vi "PeakDetect_FilterMinimumPeakWidth.vi"(6 "minimumPeakWidth":dbl format="%#_13g", 8 "Error In":errorcluster, 11 "Peak Info In":T1[](array[typedef])) -> (0 "Error Out":errorcluster, 3 "Peak Info Out":T1[](array[typedef]))   [LabVIEW 2015]
uses:
  Controls/PeakInfoPresenter.ctl
panel:
  in  "MinimumSlopeToUsePeakMax":dbl format="%#_13g"
  in  "Intensities":dbl[](array[numeric])=[55.0, 56.0, 46.0, 32.0, 21.0, 37.0, 92.0, 179.0, 213.0, 312.0, 312.0, 297.0, 296.0, 224.0, 192.0, 50.0, 58.0, 96.0, 112.0, 108.0, 107.0, 117.0, 101.0, 79.0, 28.0, 242.0, 3002.0, 4321.0, 6382.0, 8039.0, 8112.0, 7467.0, 6673.0, 6730.0, 4821.0, 161.0, 116.0, 199.0, 280.0, 324.0, 385.0, 306.0, 340.0, 270.0, 209.0, 596.0, 8839.0, 15018.0, 22096.0, 27306.0, 28282.0, 26382.0, 24772.0, 19971.0, 16031.0, 677.0, 291.0, 595.0, 848.0, 1124.0, 1192.0, 1040.0, 1069.0, 767.0, 821.0, 50.0, 66.0, 105.0, 160.0, 163.0, 147.0, 163.0, 127.0, 96.0, 73.0, 9.0, 4.0, 4.0, 19.0, 10.0, 14.0, 8.0, 14.0, 7.0, 9.0, 44.0, 57.0, 86.0, 126.0, 111.0, 98.0, 79.0, 95.0, 67.0, 16.0, 19.0, 17.0, 25.0, 30.0, 39.0, 38.0, 191.0, 275.0, 254.0, 270.0, 293.0, 216.0, 219.0, 170.0, 180.0, 186.0, 212.0, 255.0, 355.0, 365.0, 354.0, 352.0, 389.0, 310.0, 272.0, 208.0, 189.0, 175.0, 203.0, 226.0, 202.0, 206.0, 278.0, 279.0, 414.0, 799.0, 1517.0, 2446.0, 3938.0, 4796.0, 5265.0, 5583.0, 5257.0, 4438.0, 3543.0, 2831.0, 1347.0, 1119.0, 1370.0, 1782.0, 1807.0, 1828.0, 2082.0, 2011.0, 2473.0, 4735.0, 8059.0, 13114.0, 21491.0, 25990.0, 28670.0, 29595.0, 29953.0, 26733.0, 21472.0, 14896.0, 7745.0, 6381.0, 7465.0, 9646.0, 10328.0, 10403.0, 10136.0, 9622.0, 7344.0, 5462.0, 2287.0, 1703.0, 2115.0, 2635.0, 3263.0, 4044.0, 5060.0, 5508.0, 6042.0, 6139.0, 6124.0, 6909.0, 7394.0, 6919.0, 6393.0, 5036.0, 5125.0, 4926.0, 3939.0, 3280.0, 2071.0, 2019.0, 1927.0, 1569.0, 1324.0, 992.0, 958.0, 880.0, 889.0, 993.0, 1241.0, 163.0, 122.0, 143.0, 189.0, 188.0, 214.0, 226.0, 254.0, 230.0, 216.0, 170.0, 164.0, 205.0, 153.0, 204.0, 137.0, 171.0, 163.0, 229.0, 313.0, 468.0, 667.0, 1041.0, 1532.0, 1899.0, 2343.0, 2797.0, 2956.0, 2591.0, 1993.0, 1475.0, 787.0, 702.0, 842.0, 1073.0, 1341.0, 1708.0, 1886.0, 2506.0, 3796.0, 5659.0, 7754.0, 13596.0, 19036.0, 25687.0, 30761.0, 35888.0, 37967.0, 35251.0, 27029.0, 21428.0, 11593.0, 9040.0, 11127.0, 13005.0, 16089.0, 18097.0, 19329.0, 19088.0, 14510.0, 10053.0, 6086.0, 4080.0, 4322.0, 4947.0, 5697.0, 6188.0, 6839.0, 6325.0, 5298.0, 3850.0, 2157.0, 1592.0, 1569.0, 1697.0, 1935.0, 1994.0, 2079.0, 2043.0, 1563.0, 1245.0, 826.0, 516.0, 585.0, 620.0, 609.0, 625.0, 651.0, 677.0, 707.0, 761.0, 879.0, 1091.0, 1597.0, 1813.0, 2074.0, 2314.0, 2176.0, 2032.0, 1570.0, 1155.0, 21.0, 18.0, 5.0, 22.0, 10.0, 11.0, 23.0, 8.0, 11.0, 20.0, 14.0, 12.0, 22.0, 8.0, 12.0, 19.0, 14.0, 16.0, 9.0, 18.0, 12.0, 21.0, 16.0, 22.0, 13.0, 20.0, 13.0, 26.0, 26.0, 44.0, 30.0, 56.0, 52.0, 39.0, 33.0, 26.0, 18.0, 29.0, 34.0, 36.0, 39.0, 47.0, 55.0, 113.0, 124.0, 202.0, 279.0, 355.0, 573.0, 856.0, 1150.0, 1298.0, 1700.0, 1791.0, 1294.0, 1052.0, 874.0, 526.0, 667.0, 865.0, 992.0, 1286.0, 1427.0, 1381.0, 1239.0, 962.0, 662.0, 386.0, 392.0, 452.0, 513.0, 627.0, 706.0, 779.0, 523.0, 425.0, 309.0, 188.0, 172.0, 182.0, 179.0, 207.0, 285.0, 246.0, 231.0, 183.0, 112.0, 65.0, 58.0, 81.0, 73.0, 95.0, 110.0, 112.0, 67.0, 78.0, 79.0, 70.0, 78.0, 92.0, 108.0, 43.0, 40.0, 52.0, 32.0, 53.0, 51.0, 37.0, 35.0, 43.0, 33.0, 39.0, 48.0, 62.0, 38.0, 40.0, 31.0, 42.0, 31.0, 47.0, 41.0, 41.0, 46.0, 49.0, 59.0, 49.0, 56.0, 66.0, 49.0, 57.0, 78.0, 107.0, 139.0, 196.0, 263.0, 350.0, 506.0, 639.0, 850.0, 963.0, 1256.0, 1355.0, 1989.0, 2163.0, 2256.0, 2168.0, 2097.0, 1936.0, 1771.0, 1572.0, 1549.0, 1669.0, 1962.0, 1928.0, 2150.0, 2282.0, 1774.0, 1693.0, 1455.0, 1325.0, 1034.0, 984.0, 993.0, 1120.0, 1284.0, 1002.0, 1042.0, 931.0, 781.0, 614.0, 482.0, 424.0, 448.0, 432.0, 435.0, 521.0, 427.0, 389.0, 344.0, 261.0, 187.0, 173.0, 188.0, 218.0, 209.0, 195.0, 185.0, 181.0, 196.0, 212.0, 193.0, 240.0, 203.0, 266.0, 287.0, 280.0, 229.0, 230.0, 207.0, 196.0, 189.0, 180.0, 4.0, 10.0, 7.0, 13.0, 5.0, 15.0, 7.0, 3.0, 13.0, 8.0, 7.0, 8.0, 4.0, 12.0, 11.0, 4.0, 4.0, 11.0, 4.0, 6.0, 8.0, 1.0, 9.0, 11.0, 9.0, 7.0, 8.0, 16.0, 10.0, 13.0, 4.0, 6.0, 10.0, 10.0, 11.0, 15.0, 7.0, 9.0, 6.0, 7.0, 8.0, 16.0, 6.0, 12.0, 7.0, 16.0, 22.0, 63.0, 99.0, 111.0, 172.0, 250.0, 327.0, 379.0, 389.0, 354.0, 296.0, 269.0, 251.0, 177.0, 211.0, 221.0, 341.0, 372.0, 363.0, 332.0, 304.0, 314.0, 240.0, 145.0, 137.0, 169.0, 201.0, 238.0, 259.0, 183.0, 200.0, 192.0, 92.0, 77.0, 60.0, 91.0, 68.0, 87.0, 129.0, 90.0, 88.0, 76.0, 59.0, 28.0, 26.0, 22.0, 36.0, 33.0, 36.0, 47.0, 33.0, 41.0, 31.0, 38.0, 29.0]
  in  "Masses":dbl[](array[numeric])=[54.0, 54.1, 54.2, 54.3, 54.4, 54.5, 54.6, 54.7, 54.8, 54.9, 55.0, 55.1, 55.2, 55.3, 55.4, 55.5, 55.6, 55.7, 55.8, 55.9, 56.0, 56.1, 56.2, 56.3, 56.4, 56.5, 56.6, 56.7, 56.8, 56.9, 57.0, 57.1, 57.2, 57.3, 57.4, 57.5, 57.6, 57.7, 57.8, 57.9, 58.0, 58.1, 58.2, 58.3, 58.4, 58.5, 58.6, 58.7, 58.8, 58.9, 59.0, 59.1, 59.2, 59.3, 59.4, 59.5, 59.6, 59.7, 59.8, 59.9, 60.0, 60.1, 60.2, 60.3, 60.4, 60.5, 60.6, 60.7, 60.8, 60.9, 61.0, 61.1, 61.2, 61.3, 61.4, 61.5, 61.6, 61.7, 61.8, 61.9, 62.0, 62.1, 62.2, 62.3, 62.4, 62.5, 62.6, 62.7, 62.8, 62.9, 63.0, 63.1, 63.2, 63.3, 63.4, 63.5, 63.6, 63.7, 63.8, 63.9, 64.0, 611.0, 611.1, 611.2, 611.3, 611.4, 611.5, 611.6, 611.7, 611.8, 611.9, 612.0, 612.1, 612.2, 612.3, 612.4, 612.5, 612.6, 612.7, 612.8, 612.9, 613.0, 613.1, 613.2, 613.3, 613.4, 613.5, 613.6, 613.7, 613.8, 613.9, 614.0, 614.1, 614.2, 614.3, 614.4, 614.5, 614.6, 614.7, 614.8, 614.9, 615.0, 615.1, 615.2, 615.3, 615.4, 615.5, 615.6, 615.7, 615.8, 615.9, 616.0, 616.1, 616.2, 616.3, 616.4, 616.5, 616.6, 616.7, 616.8, 616.9, 617.0, 617.1, 617.2, 617.3, 617.4, 617.5, 617.6, 617.7, 617.8, 617.9, 618.0, 618.1, 618.2, 618.3, 618.4, 618.5, 618.6, 618.7, 618.8, 618.9, 619.0, 619.1, 619.2, 619.3, 619.4, 619.5, 619.6, 619.7, 619.8, 619.9, 620.0, 620.1, 620.2, 620.3, 620.4, 620.5, 620.6, 620.7, 620.8, 620.9, 621.0, 902.0, 902.1, 902.2, 902.3, 902.4, 902.5, 902.6, 902.7, 902.8, 902.9, 903.0, 903.1, 903.2, 903.3, 903.4, 903.5, 903.6, 903.7, 903.8, 903.9, 904.0, 904.1, 904.2, 904.3, 904.4, 904.5, 904.6, 904.7, 904.8, 904.9, 905.0, 905.1, 905.2, 905.3, 905.4, 905.5, 905.6, 905.7, 905.8, 905.9, 906.0, 906.1, 906.2, 906.3, 906.4, 906.5, 906.6, 906.7, 906.8, 906.9, 907.0, 907.1, 907.2, 907.3, 907.4, 907.5, 907.6, 907.7, 907.8, 907.9, 908.0, 908.1, 908.2, 908.3, 908.4, 908.5, 908.6, 908.7, 908.8, 908.9, 909.0, 909.1, 909.2, 909.3, 909.4, 909.5, 909.6, 909.7, 909.8, 909.9, 910.0, 910.1, 910.2, 910.3, 910.4, 910.5, 910.6, 910.7, 910.8, 910.9, 911.0, 911.1, 911.2, 911.3, 911.4, 911.5, 911.6, 911.7, 911.8, 911.9, 912.0, 1540.0, 1540.1, 1540.2, 1540.3, 1540.4, 1540.5, 1540.6, 1540.7, 1540.8, 1540.9, 1541.0, 1541.1, 1541.2, 1541.3, 1541.4, 1541.5, 1541.6, 1541.7, 1541.8, 1541.9, 1542.0, 1542.1, 1542.2, 1542.3, 1542.4, 1542.5, 1542.6, 1542.7, 1542.8, 1542.9, 1543.0, 1543.1, 1543.2, 1543.3, 1543.4, 1543.5, 1543.6, 1543.7, 1543.8, 1543.9, 1544.0, 1544.1, 1544.2, 1544.3, 1544.4, 1544.5, 1544.6, 1544.7, 1544.8, 1544.9, 1545.0, 1545.1, 1545.2, 1545.3, 1545.4, 1545.5, 1545.6, 1545.7, 1545.8, 1545.9, 1546.0, 1546.1, 1546.2, 1546.3, 1546.4, 1546.5, 1546.6, 1546.7, 1546.8, 1546.9, 1547.0, 1547.1, 1547.2, 1547.3, 1547.4, 1547.5, 1547.6, 1547.7, 1547.8, 1547.9, 1548.0, 1548.1, 1548.2, 1548.3, 1548.4, 1548.5, 1548.6, 1548.7, 1548.8, 1548.9, 1549.0, 1549.1, 1549.2, 1549.3, 1549.4, 1549.5, 1549.6, 1549.7, 1549.8, 1549.9, 1550.0, 1773.0, 1773.1, 1773.2, 1773.3, 1773.4, 1773.5, 1773.6, 1773.7, 1773.8, 1773.9, 1774.0, 1774.1, 1774.2, 1774.3, 1774.4, 1774.5, 1774.6, 1774.7, 1774.8, 1774.9, 1775.0, 1775.1, 1775.2, 1775.3, 1775.4, 1775.5, 1775.6, 1775.7, 1775.8, 1775.9, 1776.0, 1776.1, 1776.2, 1776.3, 1776.4, 1776.5, 1776.6, 1776.7, 1776.8, 1776.9, 1777.0, 1777.1, 1777.2, 1777.3, 1777.4, 1777.5, 1777.6, 1777.7, 1777.8, 1777.9, 1778.0, 1778.1, 1778.2, 1778.3, 1778.4, 1778.5, 1778.6, 1778.7, 1778.8, 1778.9, 1779.0, 1779.1, 1779.2, 1779.3, 1779.4, 1779.5, 1779.6, 1779.7, 1779.8, 1779.9, 1780.0, 1780.1, 1780.2, 1780.3, 1780.4, 1780.5, 1780.6, 1780.7, 1780.8, 1780.9, 1781.0, 1781.1, 1781.2, 1781.3, 1781.4, 1781.5, 1781.6, 1781.7, 1781.8, 1781.9, 1782.0, 1782.1, 1782.2, 1782.3, 1782.4, 1782.5, 1782.6, 1782.7, 1782.8, 1782.9, 1783.0, 1830.0, 1830.1, 1830.2, 1830.3, 1830.4, 1830.5, 1830.6, 1830.7, 1830.8, 1830.9, 1831.0, 1831.1, 1831.2, 1831.3, 1831.4, 1831.5, 1831.6, 1831.7, 1831.8, 1831.9, 1832.0, 1832.1, 1832.2, 1832.3, 1832.4, 1832.5, 1832.6, 1832.7, 1832.8, 1832.9, 1833.0, 1833.1, 1833.2, 1833.3, 1833.4, 1833.5, 1833.6, 1833.7, 1833.8, 1833.9, 1834.0, 1834.1, 1834.2, 1834.3, 1834.4, 1834.5, 1834.6, 1834.7, 1834.8, 1834.9, 1835.0, 1835.1, 1835.2, 1835.3, 1835.4, 1835.5, 1835.6, 1835.7, 1835.8, 1835.9, 1836.0, 1836.1, 1836.2, 1836.3, 1836.4, 1836.5, 1836.6, 1836.7, 1836.8, 1836.9, 1837.0, 1837.1, 1837.2, 1837.3, 1837.4, 1837.5, 1837.6, 1837.7, 1837.8, 1837.9, 1838.0, 1838.1, 1838.2, 1838.3, 1838.4, 1838.5, 1838.6, 1838.7, 1838.8, 1838.9, 1839.0, 1839.1, 1839.2, 1839.3, 1839.4, 1839.5, 1839.6, 1839.7, 1839.8, 1839.9, 1840.0]
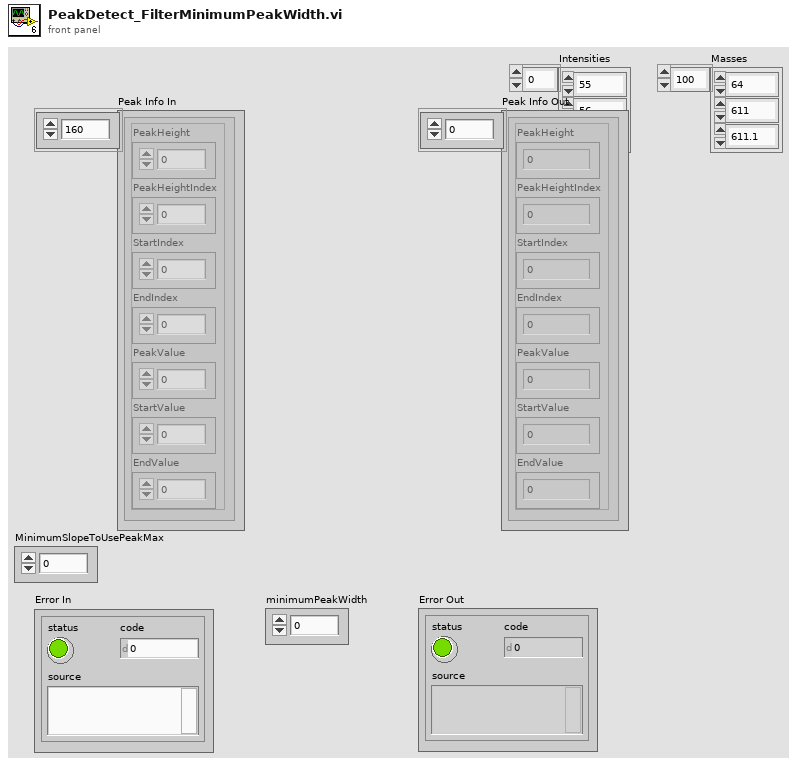
[diagram p1: front panel]
types:
  T1 = typedef "PeakInfoPresenter.ctl" = cluster{"PeakHeight":dbl, "PeakHeightIndex":dbl, "StartIndex":dbl, "EndIndex":dbl, "PeakValue":dbl, "StartValue":dbl, "EndValue":dbl}
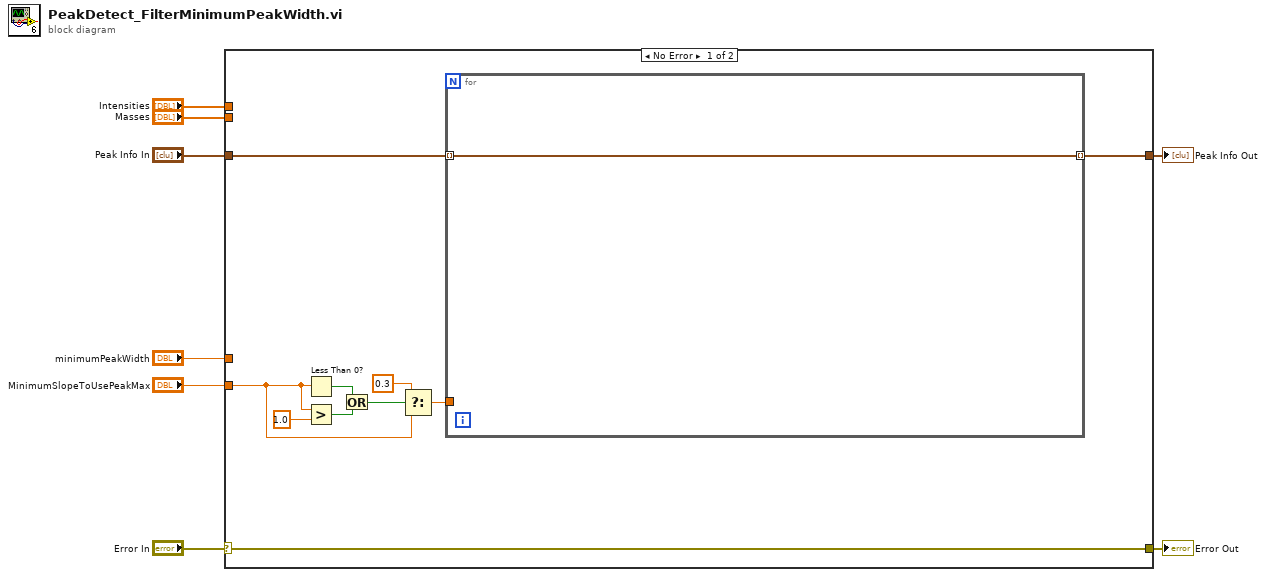
[diagram p0: block diagram]
diagram:
  n1 = case shown="No Error" "Error In" {
    selector: "Error In" -> [w18 w21]
    tunnel: [w18 w21] -> w7
    tunnel: "Peak Info In" -> [w10 w20]
    tunnel: [w11 w20] -> w5
    tunnel: "Intensities" -> [_ _]
    tunnel: "Masses" -> [_ _]
    tunnel: "minimumPeakWidth" -> [_ _]
    tunnel: "MinimumSlopeToUsePeakMax" -> [w12 _]
    frame No Error {
      n2 = Less Than 0?(x=w12) -> (x < 0?=w16:bool)
      n3 = Greater?(x=w12, y=1.0) -> (0:w15:bool)
      n4 = Or(x=w16, y=w15) -> (x .or. y?=w14:bool)
      n5 = Select(t=0.3, s=w14, f=w12) -> (s? t:f=w9:dbl)
      n6 = for {
        tunnel: [w19] -> w11 mode=indexing
        tunnel: w10 -> [w19] mode=indexing
        tunnel: w9 -> [_]
      }
    }
    frame Error {
    }
  }
  "Error Out" <- w7
  "Peak Info Out" <- w5
